vi "Autonomous Independent.vi"() -> ()   [LabVIEW 2012]
doc: "This VI is called when autonomous begins, and will automatically be terminated when autonomous ends. You can carry out timed or sensor driven robot movement independently without needing to return to the caller."
uses:
  <vilib>/Rock Robotics/WPI/Solenoid/WPI_SolenoidValue.ctl
  Robot Global Data.vi
  <vilib>/Rock Robotics/WPI/RobotDrive/WPI_RobotDriveGetSetRefNum.vi
  <vilib>/Rock Robotics/WPI/Solenoid/WPI_SolenoidSetEnum.vi
  <vilib>/Rock Robotics/WPI/Joystick/WPI_JoystickGetSetRefNum.vi
  <vilib>/Rock Robotics/WPI/RobotDrive/WPI_RobotDriveArcadeDrive_Standard(NoSaturation).vi
panel:
  out "Current Movement, for debugging":T1 {"Y Joystick Value" scale=1.0..-1.0; "X Joystick Value" scale=-1.0..1.0}
  in  "Array of robot movements":T2(array[cluster]) {"Y Joystick Value" scale=1.0..-1.0; "X Joystick Value" scale=-1.0..1.0}
  # "Be sure to right-click and choose Data Operations>>Make Current Value default if you want to save the array values with the VI"
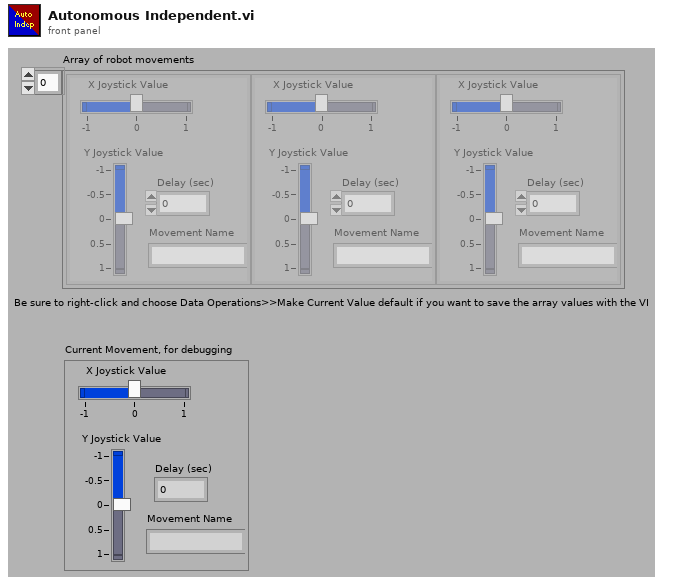
[diagram p1: front panel]
types:
  T1 = cluster{"X Joystick Value":dbl, "Y Joystick Value":dbl, "Delay (sec)":dbl, "Movement Name":string}
  T2 = cluster{"X Joystick Value":dbl, "Y Joystick Value":dbl, "Delay (sec)":dbl, "Movement Name":string}[]
  T3 = typedef "WPI_JoystickDevRef.ctl" = cluster{"Device":T4}
  T4 = typedef "WPI_JoystickDeviceEnum.ctl" = enum16{"USB 1", "USB 2", "USB 3", "USB 4", "Kinect 1", "Kinect 2"}
  T5 = cluster{"axis 1 (x)":dbl, "axis 2 (y)":dbl, "axis 3 (throttle)":dbl, "axis 4":dbl, "axis 5":dbl, "axis 6":dbl}
  T6 = typedef "WPI_SolenoidValue.ctl" = enum16{"Off", "On", "Forward", "Reverse"}
  T7 = typedef "WPI_RobotDriveDevRef.ctl" = cluster{"DevStatus":errorcluster, "Motors[]":T8[], "Square Inputs":bool, "Max Output":dbl, "Isochronous":bool}
  T8 = typedef "WPI_MotorControlDeviceRef.ctl" = cluster{"DeviceStatus":errorcluster, "Type":enum16{"PWM", "CAN"}, "PWM":cluster{"Digital Module":T9, "PWM Channel":T10, "DeadBand":T11}, "CAN":cluster{"Device Number":u8, "Control Mode":T12, "Semaphore":T13, "Max Vout":dbl}, "Invert":bool, "TransformRef":T14, "InvTransformRef":T14}
  T9 = typedef "FPGA_TypedefDigitalModule.ctl" = enum16{"Digital Module 1", "Digital Module 2"}
  T10 = typedef "FPGA_DIOPWMChannel.ctl" = enum8{"PWM 1", "PWM 2", "PWM 3", "PWM 4", "PWM 5", "PWM 6", "PWM 7", "PWM 8", "PWM 9", "PWM 10", "Invalid"}
  T11 = typedef "WPI_PWMDeadband.ctl" = cluster{"Name":string, "maxPositivePwm":i32, "minPositivePwm":i32, "centerPwm":i32, "maxNegativePwm":i32, "minNegativePwm":i32, "angularRange":u16}
  T12 = typedef "WPI_CANJaguar_ControlMode.ctl" = enum8{"Percent VBus", "Current", "Speed", "Position", "Voltage"}
  T13 = typedef "Semaphore RefNum" = refnum<k1>
  T14 = typedef "WPI_PWMTransform_ConPane.ctl" = refnum<vi>
  T15 = typedef "WPI_SolenoidDevRef.ctl" = cluster{"DevStatus":errorcluster, "Solenoid Module":T16, "Forward Solenoid Channel":T17, "Reverse Solenoid Channel":T17}
  T16 = typedef "FPGA_TypedefSolenoidModule.ctl" = enum16{"Solenoid Module 1", "Solenoid Module 2"}
  T17 = typedef "WPI_SolenoidChannel.ctl" = enum8{"Solenoid 1", "Solenoid 2", "Solenoid 3", "Solenoid 4", "Solenoid 5", "Solenoid 6", "Solenoid 7", "Solenoid 8", "Invalid"}
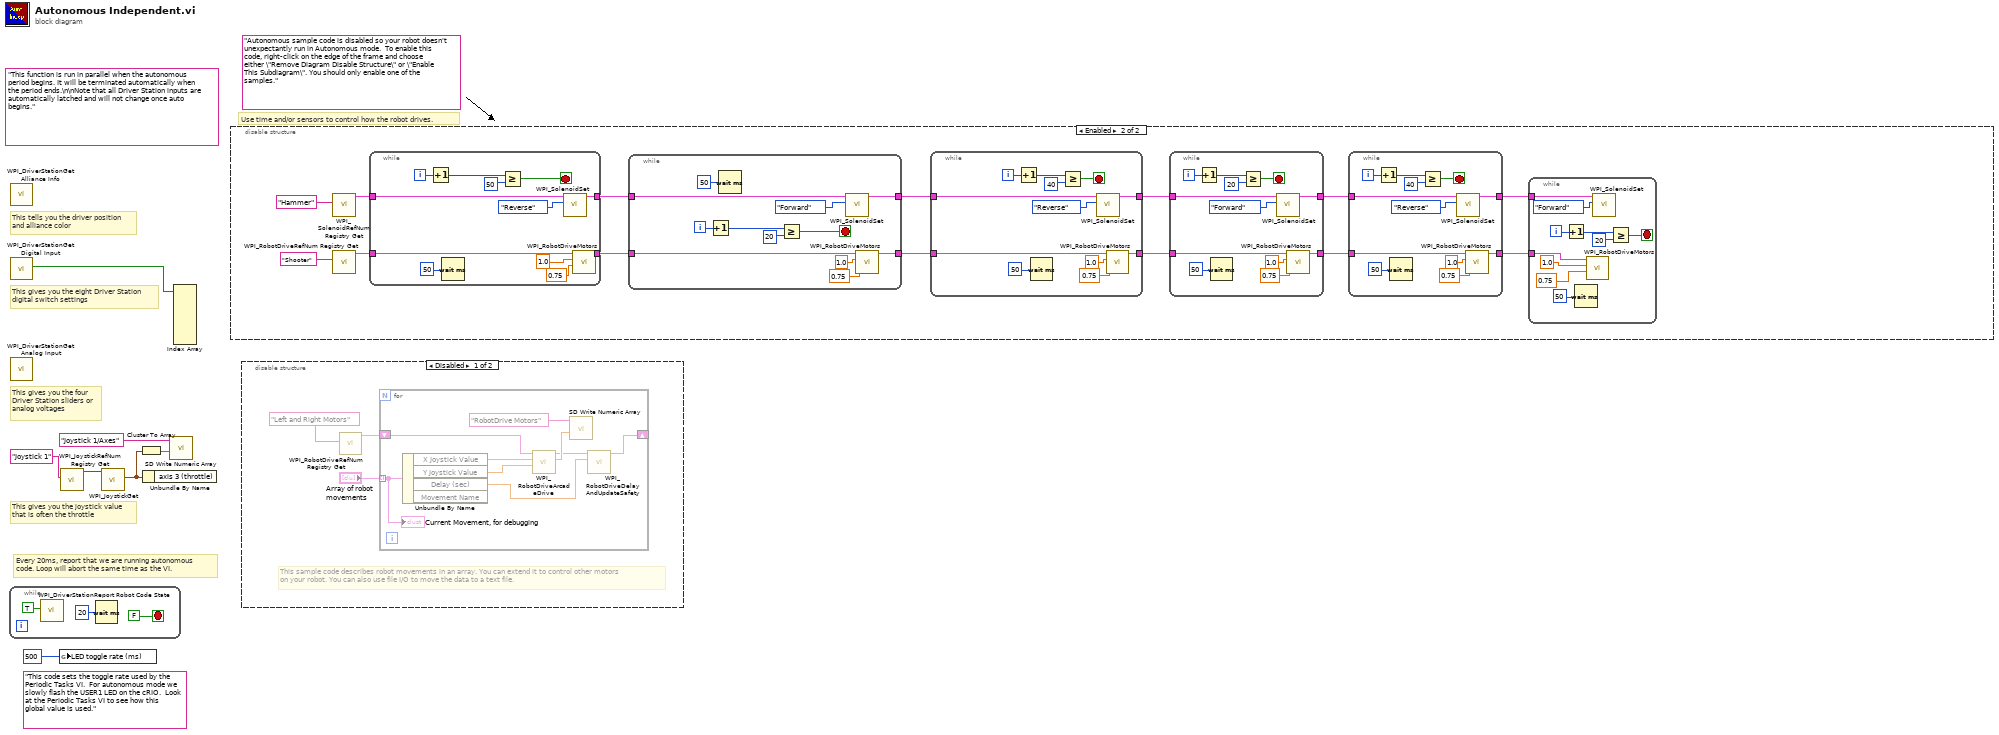
[diagram p0: block diagram]
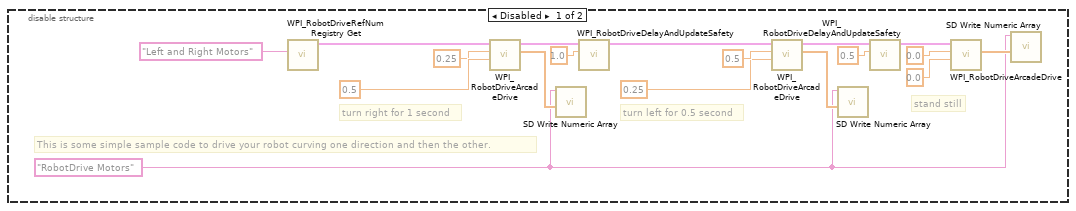
[diagram p3: hidden frame]
diagram:
  (unwired) "This code sets the toggle rate used by the Periodic Tasks VI.  For autonomous mode we slowly flash the USER1 LED on the cRIO.  Look at the Periodic Tasks VI to see how this global value is used."
  (unwired) "Autonomous sample code is disabled so your robot doesn't unexpectantly run in Autonomous mode.  To enable this code, right-click on the edge of the frame and choose either \"Remove Diagram Disable Structure\" or \"Enable This Subdiagram\". You should only enable one of the samples."
  (unwired) "This function is run in parallel when the autonomous period begins. It will be terminated automatically when the period ends.\n\nNote that all Driver Station inputs are automatically latched and will not change once auto begins."
  # "Every 20ms, report that we are running autonomous\ncode. Loop will abort the same time as the VI."
  # "This gives you the joystick value\nthat is often the throttle"
  # "Use time and/or sensors to control how the robot drives."
  # "This tells you the driver position\nand alliance color"
  # "This gives you the eight Driver Station\ndigital switch settings"
  # "This gives you the four\nDriver Station sliders or\nanalog voltages"
  n1 = while {
    stop <- FALSE stop-if-true
    n2 = call <vilib>:"WPI_DriverStationReport Robot Code State.vi"("Autonomous"=TRUE) -> ()  [unwired: 10 in, 1 out]
    n3 = Wait (ms)(milliseconds to wait=u32 20) -> ()  [unwired: 1 out]
  }
  n4 = call <vilib>:"WPI_DriverStationGet Alliance Info.vi"() -> ()  [unwired: 12 out]
  n5 = call <vilib>:"WPI_DriverStationGet Digital Input.vi"() -> ("Driver Station Digital Input (1-8)"=w7:bool[])  [unwired: 11 out]
  n6 = call <vilib>:"WPI_DriverStationGet Analog Input.vi"() -> ()  [unwired: 12 out]
  n7 = global write "Robot Global Data.vi" "LED toggle rate (ms)"(u32 500 ("LED ms toggle rate")) -> ()
  n8 = call <vilib>:"WPI_JoystickRefNum Registry Get.vi"("refnum name"="Joystick 1") -> ("JoystickDevRef"=w5:T3)  [unwired: 1 in, 9 out]
  n9 = call <vilib>:"WPI_JoystickGet.vi"("JoystickDevRef"=w5) -> ("Axes"=w2:T5)  [unwired: 1 in, 5 out]
  n10 = Cluster To Array(cluster=w2) -> (array=w3:dbl[])
  n11 = Unbundle By Name(w2) -> ()  [unwired: 1 out]
  n12 = call <vilib>:"SD Write Numeric Array.vi"("Numeric Array"=w3, "Name"="Joystick 1/Axes") -> ()  [unwired: 8 in, 2 out]
  n13 = Index Array(array=w7) -> ()  [unwired: 8 in, 8 out]
  n14 = disable-structure shown="Enabled" {
    frame Disabled {
      w11 = "RobotDrive Motors" ("Name")
      # "This is some simple sample code to drive your robot curving one direction and then the other."
      # "stand still"
      # "turn left for 0.5 second"
      # "turn right for 1 second"
      n15 = call <vilib>:"WPI_RobotDriveRefNum Registry Get.vi"("refnum name"="Left and Right Motors") -> ("RobotDriveDevRef"=w15:T7)  [unwired: 1 in, 9 out]
      n16 = call-poly <vilib>:"WPI_RobotDriveArcadeDrive.vi"("Y axis value"=0.5 ("X axis value"), "X axis value"=0.25, "RobotDriveDevRef"=w15) -> ("Motor Values"=w14:dbl[], "RobotDriveDevRef"=w22:T7)  [unwired: 1 in, 6 out]
      n17 = call <vilib>:"SD Write Numeric Array.vi"("Numeric Array"=w14, "Name"=w11) -> ()  [unwired: 8 in, 2 out]
      n18 = call <vilib>:"WPI_RobotDriveDelayAndUpdateSafety.vi"("Delay (s)"=1.0, "RobotDriveDevRef"=w22) -> ("RobotDriveDevRef 2"=w21:T7)  [unwired: 8 in, 1 out]
      n19 = call-poly <vilib>:"WPI_RobotDriveArcadeDrive.vi"("Y axis value"=0.25 ("X axis value"), "X axis value"=0.5, "RobotDriveDevRef"=w21) -> ("Motor Values"=w13:dbl[], "RobotDriveDevRef"=w20:T7)  [unwired: 1 in, 6 out]
      n20 = call <vilib>:"SD Write Numeric Array.vi"("Numeric Array"=w13, "Name"=w11) -> ()  [unwired: 8 in, 2 out]
      n21 = call <vilib>:"WPI_RobotDriveDelayAndUpdateSafety.vi"("Delay (s)"=0.5, "RobotDriveDevRef"=w20) -> ("RobotDriveDevRef 2"=w19:T7)  [unwired: 8 in, 1 out]
      n22 = call-poly <vilib>:"WPI_RobotDriveArcadeDrive.vi"("Y axis value"=0.0 ("X axis value"), "X axis value"=0.0, "RobotDriveDevRef"=w19) -> ("Motor Values"=w12:dbl[])  [unwired: 1 in, 7 out]
      n23 = call <vilib>:"SD Write Numeric Array.vi"("Numeric Array"=w12, "Name"=w11) -> ()  [unwired: 8 in, 2 out]
    }
    frame Enabled {
      n24 = call <vilib>:"WPI_SolenoidRefNum Registry Get.vi"("refnum name"="Hammer") -> ("SolenoidDevRef"=w39:T15)  [unwired: 9 in, 1 out]
      n25 = call <vilib>:"WPI_RobotDriveRefNum Registry Get.vi"("refnum name"="Shooter") -> ("RobotDriveDevRef"=w40:T7)  [unwired: 1 in, 9 out]
      n26 = while {
        tunnel: w40 -> [w110]
        tunnel: w39 -> [w109]
        tunnel: [w104] -> w38
        tunnel: [w103] -> w37
        i -> [w105]
        stop <- w106 stop-if-true
        n27 = Increment(x=w105) -> (x+1=w107:i32)
        n28 = Wait (ms)(milliseconds to wait=u32 50) -> ()  [unwired: 1 out]
        n29 = Greater Or Equal?(x=w107, y=50) -> (x >= y?=w106:bool)
        n30 = call-poly <vilib>:"WPI_SolenoidSet.vi"("Value"=WPI_SolenoidValue."Reverse", "SolenoidDevRef"=w109) -> ("SolenoidDevRef"=w103:T15)  [unwired: 8 in, 1 out]
        n31 = call <vilib>:"WPI_RobotDriveMotors.vi"("RightSpeed"=0.75, "LeftSpeed"=1.0 ("X axis value"), "RobotDriveDevRef"=w110) -> ("RobotDriveDevRef"=w104:T7)  [unwired: 6 in, 2 out]
      }
      n32 = while {
        tunnel: w38 -> [w100]
        tunnel: w37 -> [w99]
        tunnel: [w91] -> w36
        tunnel: [w90] -> w35
        i -> [w93]
        stop <- w94 stop-if-true
        n33 = Increment(x=w93) -> (x+1=w97:i32)
        n34 = Wait (ms)(milliseconds to wait=u32 50) -> ()  [unwired: 1 out]
        n35 = Greater Or Equal?(x=w97, y=20) -> (x >= y?=w94:bool)
        n36 = call-poly <vilib>:"WPI_SolenoidSet.vi"("Value"=WPI_SolenoidValue."Forward", "SolenoidDevRef"=w99) -> ("SolenoidDevRef"=w90:T15)  [unwired: 8 in, 1 out]
        n37 = call <vilib>:"WPI_RobotDriveMotors.vi"("RightSpeed"=0.75, "LeftSpeed"=1.0, "RobotDriveDevRef"=w100) -> ("RobotDriveDevRef"=w91:T7)  [unwired: 6 in, 2 out]
      }
      n38 = while {
        tunnel: w36 -> [w88]
        tunnel: w35 -> [w87]
        tunnel: [w79] -> w34
        tunnel: [w78] -> w33
        i -> [w81]
        stop <- w82 stop-if-true
        n39 = Increment(x=w81) -> (x+1=w85:i32)
        n40 = Wait (ms)(milliseconds to wait=u32 50) -> ()  [unwired: 1 out]
        n41 = Greater Or Equal?(x=w85, y=40) -> (x >= y?=w82:bool)
        n42 = call-poly <vilib>:"WPI_SolenoidSet.vi"("Value"=WPI_SolenoidValue."Reverse", "SolenoidDevRef"=w87) -> ("SolenoidDevRef"=w78:T15)  [unwired: 8 in, 1 out]
        n43 = call <vilib>:"WPI_RobotDriveMotors.vi"("RightSpeed"=0.75, "LeftSpeed"=1.0, "RobotDriveDevRef"=w88) -> ("RobotDriveDevRef"=w79:T7)  [unwired: 6 in, 2 out]
      }
      n44 = while {
        tunnel: w34 -> [w76]
        tunnel: w33 -> [w75]
        tunnel: [w67] -> w32
        tunnel: [w66] -> w31
        i -> [w69]
        stop <- w70 stop-if-true
        n45 = Increment(x=w69) -> (x+1=w73:i32)
        n46 = Wait (ms)(milliseconds to wait=u32 50) -> ()  [unwired: 1 out]
        n47 = Greater Or Equal?(x=w73, y=20) -> (x >= y?=w70:bool)
        n48 = call-poly <vilib>:"WPI_SolenoidSet.vi"("Value"=WPI_SolenoidValue."Forward", "SolenoidDevRef"=w75) -> ("SolenoidDevRef"=w67:T15)  [unwired: 8 in, 1 out]
        n49 = call <vilib>:"WPI_RobotDriveMotors.vi"("RightSpeed"=0.75, "LeftSpeed"=1.0, "RobotDriveDevRef"=w76) -> ("RobotDriveDevRef"=w66:T7)  [unwired: 6 in, 2 out]
      }
      n50 = while {
        tunnel: w31 -> [w64]
        tunnel: w32 -> [w63]
        tunnel: [w55] -> w30
        tunnel: [w54] -> w29
        i -> [w57]
        stop <- w58 stop-if-true
        n51 = Increment(x=w57) -> (x+1=w61:i32)
        n52 = Wait (ms)(milliseconds to wait=u32 50) -> ()  [unwired: 1 out]
        n53 = Greater Or Equal?(x=w61, y=40) -> (x >= y?=w58:bool)
        n54 = call-poly <vilib>:"WPI_SolenoidSet.vi"("Value"=WPI_SolenoidValue."Reverse", "SolenoidDevRef"=w63) -> ("SolenoidDevRef"=w54:T15)  [unwired: 8 in, 1 out]
        n55 = call <vilib>:"WPI_RobotDriveMotors.vi"("RightSpeed"=0.75, "LeftSpeed"=1.0, "RobotDriveDevRef"=w64) -> ("RobotDriveDevRef"=w55:T7)  [unwired: 6 in, 2 out]
      }
      n56 = while {
        tunnel: w30 -> [w52]
        tunnel: w29 -> [w51]
        i -> [w45]
        stop <- w46 stop-if-true
        n57 = Increment(x=w45) -> (x+1=w49:i32)
        n58 = Wait (ms)(milliseconds to wait=u32 50) -> ()  [unwired: 1 out]
        n59 = call <vilib>:"WPI_RobotDriveMotors.vi"("RightSpeed"=0.75, "LeftSpeed"=1.0, "RobotDriveDevRef"=w52) -> ()  [unwired: 6 in, 3 out]
        n60 = call-poly <vilib>:"WPI_SolenoidSet.vi"("Value"=WPI_SolenoidValue."Forward", "SolenoidDevRef"=w51) -> ()  [unwired: 8 in, 2 out]
        n61 = Greater Or Equal?(x=w49, y=20) -> (x >= y?=w46:bool)
      }
    }
  }
  n62 = disable-structure shown="Disabled" {
    frame Disabled {
      # "This sample code describes robot movements in an array. You can extend it to control other motors\non your robot. You can also use file I/O to move the data to a text file."
      n63 = call <vilib>:"WPI_RobotDriveRefNum Registry Get.vi"("refnum name"="Left and Right Motors") -> ("RobotDriveDevRef"=w114:T7)  [unwired: 1 in, 9 out]
      n64 = for {
        shift-right: [w120] -> _
        shift-left: w114 -> [w121]
        tunnel: "Array of robot movements" -> [w116] mode=indexing
        n65 = Unbundle By Name(w116) -> ("X Joystick Value"=w119:dbl, "Y Joystick Value"=w118:dbl, "Delay (sec)"=w117:dbl)  [unwired: 1 out]
        n66 = call-poly <vilib>:"WPI_RobotDriveArcadeDrive.vi"("Y axis value"=w118, "X axis value"=w119, "RobotDriveDevRef"=w121) -> ("Motor Values"=w123:dbl[], "RobotDriveDevRef"=w122:T7)  [unwired: 1 in, 6 out]
        n67 = call <vilib>:"SD Write Numeric Array.vi"("Numeric Array"=w123, "Name"="RobotDrive Motors") -> ()  [unwired: 8 in, 2 out]
        n68 = call <vilib>:"WPI_RobotDriveDelayAndUpdateSafety.vi"("Delay (s)"=w117, "RobotDriveDevRef"=w122) -> ("RobotDriveDevRef 2"=w120:T7)  [unwired: 8 in, 1 out]
        "Current Movement, for debugging" <- w116
      }
    }
    frame Enabled {
    }
  }
